vi "add_line_feed.vi"(1 "Input string":string) -> (0 "Output string":string)   [LabVIEW 2017]
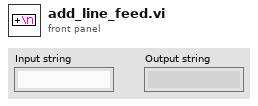
[diagram p1: front panel]
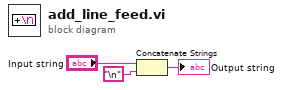
[diagram p0: block diagram]
diagram:
  n1 = Concatenate Strings("Input string", "\n") -> (→"Output string":string)
